vi "Rumble.vi"(10 "pVibration":cluster{"wLeftMotorSpeed":u16}, 11 "dwUserIndex":u32) -> (2 "pVibration out":cluster{"wLeftMotorSpeed":u16}, 3 "function return":u32)   [LabVIEW 2014]
uses:
  XInput9_1_0.dll
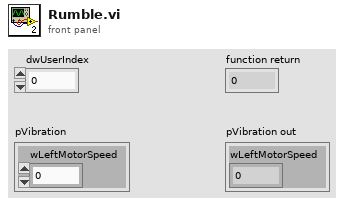
[diagram p1: front panel]
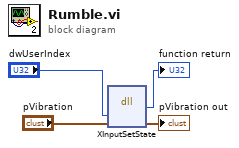
[diagram p0: block diagram]
diagram:
  n1 = dll-call lib="XInput9_1_0.*" fn="XInputSetState"("dwUserIndex"="dwUserIndex", "pVibration"="pVibration") -> (→"function return":u32, "pVibration"=→"pVibration out":cluster{"wLeftMotorSpeed":u16})  [unwired: 4 in, 2 out]
